vi "Dvr Close Ref.vi"(8 "Error In":errorcluster, 11 "Data Value Reference In":refnum<data-value>) -> (0 "Error Out":errorcluster, 3 "Data Value Reference Out":refnum<data-value>)   [LabVIEW 2021, in "Calculator.lvlib" / "NumericOperation.lvclass"]
doc: "This VI acts as a wrapper VI which calls an overriding method CloseRefnum of the corresponding class based on the Data Value Reference."
uses:
  NumericOperation.lvclass
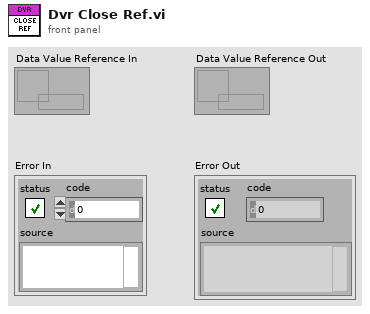
[diagram p1: front panel]
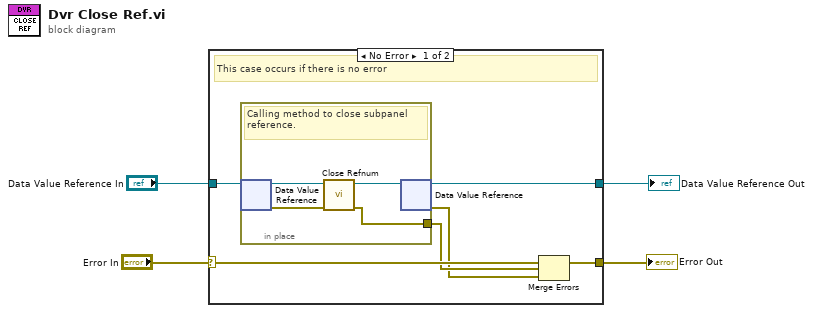
[diagram p0: block diagram]
diagram:
  n1 = case shown="No Error" "Error In" {
    selector: "Error In" -> [w8 w16]
    tunnel: [w5 w16] -> w3
    tunnel: "Data Value Reference In" -> [w10 w15]
    tunnel: [w9 w15] -> w1
    frame No Error {
      # "This case occurs if there is no error"
      n2 = in-place {
        in-place-border: [w11] -> w7
        # "Calling method to close subpanel reference."
        n3 = in-place-dvr #1(w10) -> (w14:refnum<class "NumericOperation.lvclass">, w12:errorcluster)
        n4 = call-dynamic "Close Refnum.vi"("Error In"=w12, "NumericOperation in"=w14) -> ("Error Out"=w11:errorcluster, "NumericOperation out"=w13:refnum<class "NumericOperation.lvclass">)  [unwired: 8 in]
        n5 = in-place-dvr #1(w13) -> (w9:refnum<data-value>, w6:errorcluster)
      }
      n6 = Merge Errors(w8, w7, w6) -> (w5:errorcluster)
    }
    frame Error {
      # "This case occurs if there is any error."
    }
  }
  "Error Out" <- w3
  "Data Value Reference Out" <- w1
